vi "onValueChange.vi"(8 "error in (no error)":errorcluster, 11 "Filled Text Fields Actor in":refnum<class "Filled Text Fields Actor.lvclass">) -> (0 "error out":errorcluster, 3 "Filled Text Fields Actor out":refnum<class "Filled Text Fields Actor.lvclass">)   [LabVIEW 2017, in "Filled Text Fields Actor.lvlib" / "Filled Text Fields Actor.lvclass"]
uses:
  Filled Text Fields Actor.lvclass
  C:/Program Files (x86)/National Instruments/LabVIEW 2017/vi.lib/ActorFramework/Actor/Actor.lvclass
  <vilib>/ActorFramework/Actor/Actor.lvclass/Actor.ctl
  <vilib>/ActorFramework/Message Enqueuer/Message Enqueuer.lvclass/Message Enqueuer.ctl
  Filled Text Fields Actor.lvclass/Filled Text Fields Actor.ctl
  <vilib>/ActorFramework/Message Enqueuer/Init from Existing Queue.vi
  <vilib>/ActorFramework/Message Enqueuer/Message Enqueuer.lvclass
  Filled Text Fields Actor Messages/onMouseDown Msg/onMouseDown Msg.lvclass
  <vilib>/ActorFramework/Actor/Actor.lvclass
  Filled Text Fields Actor Messages/onLeave Msg/onLeave Msg.lvclass
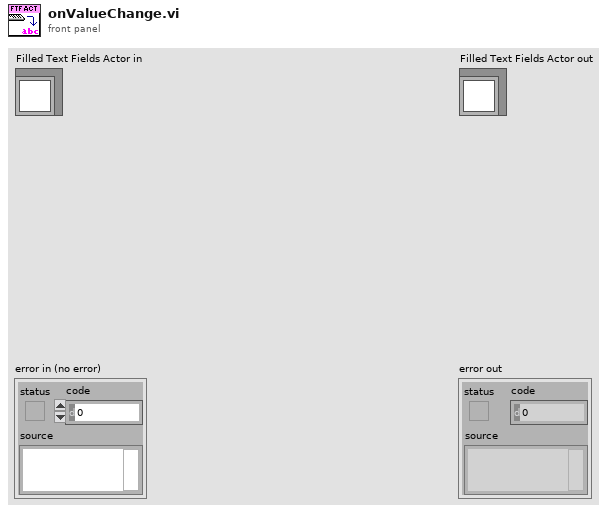
[diagram p1: front panel]
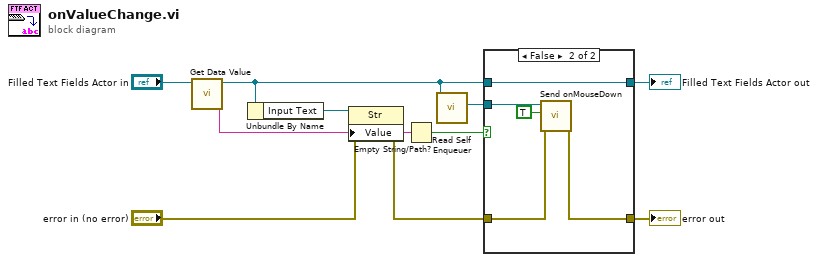
[diagram p0: block diagram]
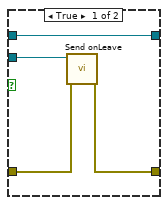
[diagram p2: hidden frame]
diagram:
  n1 = call "Get Data Value.vi"("Filled Text Fields Actor in"="Filled Text Fields Actor in") -> ("Value"=w7:string, "Filled Text Fields Actor out"=w2:refnum<class "Filled Text Fields Actor.lvclass">)  [unwired: 9 in]
  n2 = Unbundle By Name(w2) -> ("Input Text"=w9:refnum<vi>)
  n3 = property class="Str"(reference=w9, error in="error in (no error)", "Value"=w7) -> (error out=w5:errorcluster)  [unwired: 1 out]
  n4 = Empty String/Path?(string/path=w7) -> (empty?=w6:bool)
  n5 = call <vilib>:"Read Self Enqueuer.vi"("Actor"=w2) -> ("Self Enqueuer"=w1:refnum<class "Message Enqueuer.lvclass">)  [unwired: 10 in]
  n6 = case shown="False" w6 {
    tunnel: w5 -> [w12 w17]
    tunnel: w2 -> [w14 w19]
    tunnel: [w14 w19] -> w4
    tunnel: [w11 w16] -> w3
    tunnel: w1 -> [w13 w18]
    frame True {
      n7 = call "Send onLeave.vi"("error in (no error)"=w12, "Message Enqueuer in"=w13) -> ("error out"=w11:errorcluster)  [unwired: 8 in, 1 out]
    }
    frame False {
      n8 = call "Send onMouseDown.vi"("error in (no error)"=w17, "Invert"=TRUE, "Message Enqueuer in"=w18) -> ("error out"=w16:errorcluster)  [unwired: 7 in, 1 out]
    }
  }
  "error out" <- w3
  "Filled Text Fields Actor out" <- w4
